vi "PXI-Dequeue AI Data.vi"(11 "error in (no error)":errorcluster) -> (10 "AI Waveforms":dbl[][](array[numeric]), 15 "error out":errorcluster)   [LabVIEW 2020]
uses:
  DAQ Engine VIs/PXI Globals.vi
panel:
  out "Time":i32
  in  "queue out":refnum<queue>
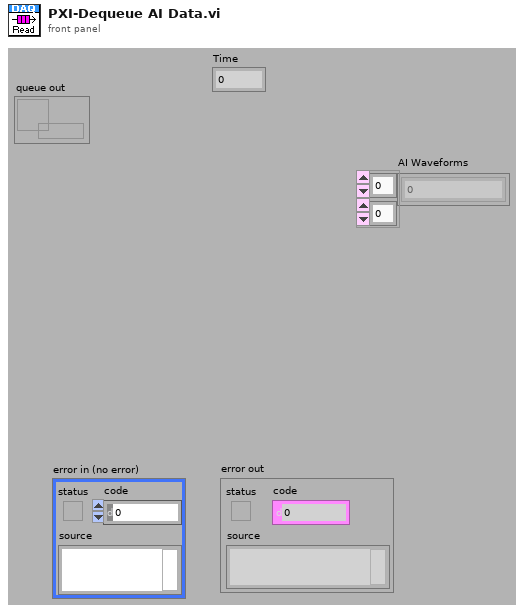
[diagram p1: front panel]
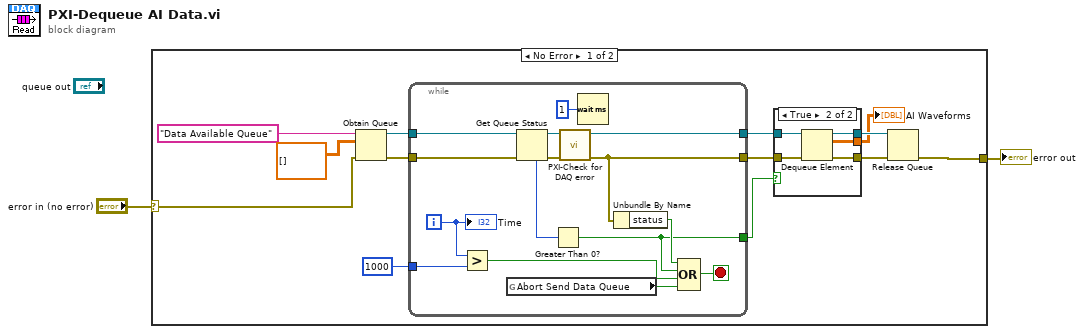
[diagram p0: block diagram]
diagram:
  n1 = case shown="No Error" "error in (no error)" {
    selector: "error in (no error)" -> [w11 w37]
    tunnel: [w15 w37] -> w2
    frame No Error {
      n2 = Obtain Queue(name (unnamed)="Data Available Queue", element data type=dbl[][] [] ("AI Waveforms 2"), error in (no error)=w11) -> (queue out=w12:refnum<queue>, error out=w10:errorcluster)  [unwired: 2 in, 1 out]
      n3 = while {
        tunnel: [w32] -> w8
        tunnel: w12 -> [w36]
        tunnel: [w29] -> w6
        tunnel: w10 -> [w30]
        tunnel: 1000 ("timeout in ms (-1)") -> [w27]
        tunnel: [w24] -> w4
        i -> [w25]
        stop <- w34 stop-if-true
        n4 = Greater?(x=w25, y=w27) -> (0:w26:bool)
        n5 = global read "PXI Globals.vi" "Abort Send Data Queue"() -> (w35:bool)
        n6 = Get Queue Status(queue=w36, error in (no error)=w30) -> (queue out=w29:refnum<queue>, error out=w28:errorcluster, # elements in queue=w23:i32)  [unwired: 1 in, 5 out]
        n7 = Greater Than 0?(x=w23) -> (x > 0?=w24:bool)
        n8 = call "PXI-Check for DAQ error.vi"("error in (no error)"=w28) -> ("error out"=w32:errorcluster)  [unwired: 14 in]
        n9 = Wait (ms)(milliseconds to wait=u32 1) -> ()  [unwired: 1 out]
        n10 = Unbundle By Name(w32) -> ("status"=w33:bool)
        n11 = Compound Arithmetic op=OR(w33, w24, w26, w35) -> (w34:bool)
        "Time" <- w25
      }
      n12 = case shown="True" w4 {
        tunnel: w8 -> [w16 w22]
        tunnel: [w16 w21] -> w7
        tunnel: w6 -> [w17 w20]
        tunnel: [w17 w19] -> w5
        tunnel: [_ w18] -> w3
        frame False {
        }
        frame True {
          n13 = Dequeue Element(queue=w20, error in (no error)=w22) -> (queue out=w19:refnum<queue>, element=w18:dbl[][], error out=w21:errorcluster)  [unwired: 1 in, 1 out]
        }
      }
      "AI Waveforms" <- w3
      n14 = Release Queue(queue=w5, error in (no error)=w7) -> (error out=w15:errorcluster)  [unwired: 1 in, 2 out]
    }
    frame Error {
    }
  }
  "error out" <- w2
